vi "get experiment lines.vi"(8 "error in (no error)":errorcluster) -> (0 "error out":errorcluster, 3 "Output Array":string[](array[string]))   [LabVIEW 2020]
uses:
  <userlib>/_OpenG.lib/array/array.llb/Remove Duplicates from 1D Array (String)__ogtk.vi
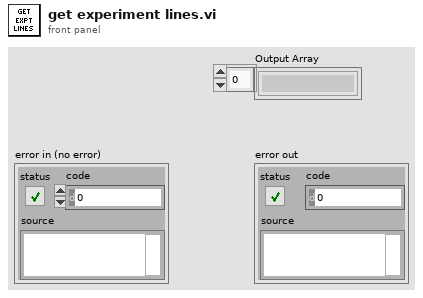
[diagram p1: front panel]
types:
  T1 = typedef "mysql_authentication.ctl" = cluster{"User":string, "Password":string, "Database":string}
  T2 = cluster{"Port":u16, "IP Address":string, "Authentication":T1}
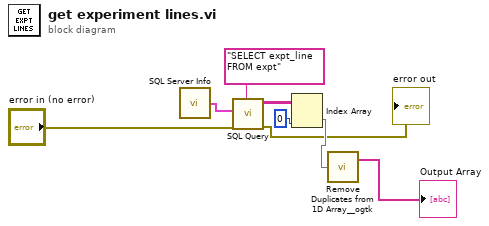
[diagram p0: block diagram]
diagram:
  n1 = call "SQL Server Info.vi"() -> ("SQL Server Info"=w3:T2)
  n2 = call "SQL Query.vi"("error in (no error)"="error in (no error)", "SQL Server Info"=w3, "Query"="SELECT expt_line FROM expt") -> ("error out"=→"error out":errorcluster, "data"=w2:string[][])  [unwired: 7 in]
  n3 = Index Array(array=w2, index (col)=0 ("disabled index (col)")) -> (element=w7:string[])  [unwired: 1 in]
  n4 = call-poly <userlib>:"Remove Duplicates from 1D Array__ogtk.vi"("Input Array"=w7) -> ("Output Array"=→"Output Array":string[])  [unwired: 1 out]
